vi "SR830 set reference mode.vi"(8 "error in (no error)":errorcluster, 10 "reference mode":enum16{"external", "internal"}(ring), 11 "VISA resource name":refnum<visa-resource-name>) -> (0 "error out":errorcluster, 3 "VISA resource name out":refnum<visa-resource-name>)   [LabVIEW 2009, in "SR830.lvlib"]
doc: "Sets the current reference mode (internal or external) of the lock-in amplifier."
uses:
  SR830.lvlib
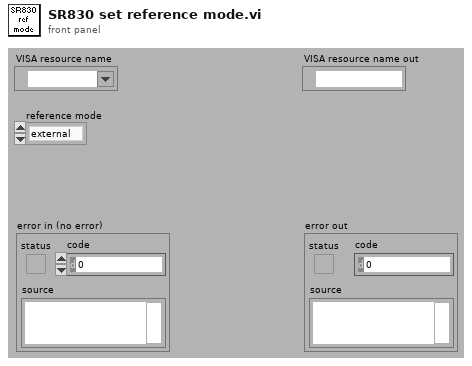
[diagram p1: front panel]
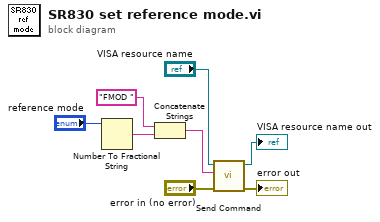
[diagram p0: block diagram]
diagram:
  n1 = Number To Fractional String(number="reference mode") -> (F-format string=w6:string)  [unwired: 3 out]
  n2 = Concatenate Strings("FMOD " ("write buffer"), w6) -> (w3:string)
  n3 = call "Send Command.vi"("error in (no error)"="error in (no error)", "write buffer"=w3, "VISA resource name"="VISA resource name") -> ("error out"=→"error out":errorcluster, "VISA resource name out"=→"VISA resource name out":refnum<visa-resource-name>)  [unwired: 7 in]
